vi "Offset_Gain.vi"() -> ()   [LabVIEW 2019]
uses:
  <userlib>/_TI-LA/Instr Drivers/Signal Generator/33XXX/Driver/EasyIO/Typedef/33XXX Standard Waveform Configuration.ctl
  <userlib>/_TI-LA/Instr Drivers/Signal Generator/33XXX/Driver/EasyIO/Typedef/33XXX Waveform Function.ctl
  <userlib>/_TI-LA/Instr Drivers/Signal Generator/33XXX/Driver/EasyIO/Typedef/33XXX Waveform Unit.ctl
  <userlib>/_TI-LA/Instr Drivers/Signal Generator/33XXX/Driver/EasyIO/Typedef/33XXX Output Load.ctl
  <userlib>/_TI-LA/Instr Drivers/Signal Generator/33XXX/Driver/EasyIO/Typedef/33XXX Output Load Termination.ctl
  <userlib>/_TI-LA/Instr Drivers/Signal Generator/33XXX/Driver/33XXX.lvlib
  <userlib>/_TI-LA/Instr Drivers/Signal Generator/33XXX/Modules/33XXX Modules.lvlib
  <vilib>/Analysis/NI_AALPro.lvlib
panel:
  out "intercept":dbl
  out "slope":dbl
  out "Array":dbl[](array[numeric])
  in  "lv_scomp":u16=8
  in  "lv_ref_vol":u16
  in  "lv_ref_sel":u16
  in  "Standard Waveform Configuration":T1={"Frequency (Hz)"=1000.0, "Waveform Function"=1, "DC Offset (V)"=0.0, "Unit"=0, "Amplitude (V)"=1.0, "Duty cycle (%)"=50.0} {"Duty cycle (%)" min=0.002 max=99.999 step=0.001 format="%.3p"; "Amplitude (V)" min=0.001 max=20.0 format="%#_6p"; "Unit" items=["Vpp", "Vrms", "dB"]; "DC Offset (V)" min=-10.0 max=10.0 format="%#_6p"; "Waveform Function" items=["DC", "Sine", "Square", "Triangle", "Ramp", "Pulse", "Noise", "Sinc", "Negative Ramp", "Exponential Rise", "Exponential Fall", "Cardiac"]; "Frequency (Hz)" min=1e-06 max=80000000.0 format="%#_6p"}
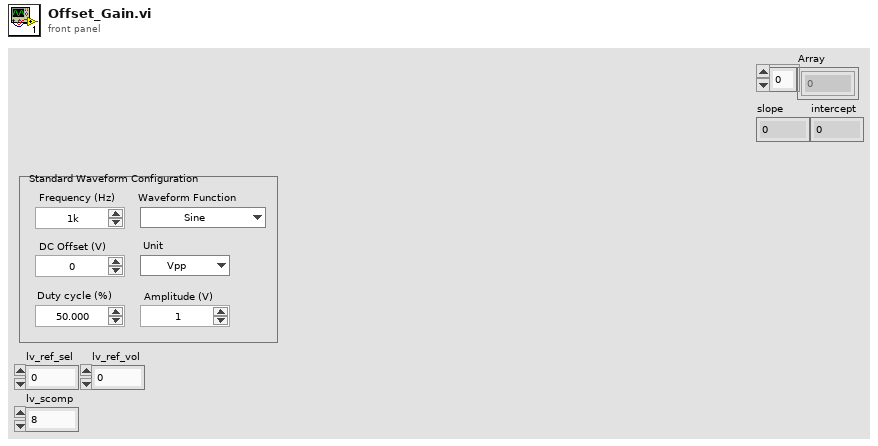
[diagram p1: front panel]
types:
  T1 = typedef "33XXX.lvlib/33XXX Standard Waveform Configuration.ctl" = cluster{"Frequency (Hz)":dbl, "Waveform Function":T2, "DC Offset (V)":dbl, "Unit":T3, "Amplitude (V)":dbl, "Duty cycle (%)":dbl}
  T2 = typedef "33XXX.lvlib/33XXX Waveform Function.ctl" = u16
  T3 = typedef "33XXX.lvlib/33XXX Waveform Unit.ctl" = u16
  T4 = typedef "33XXX.lvlib/33XXX Output Load.ctl" = cluster{"Output Load Impedence":T5, "Load value (ohms)":dbl}
  T5 = typedef "33XXX.lvlib/33XXX Output Load Termination.ctl" = enum16{"50 Ohms", "High Z", "User Defined"}
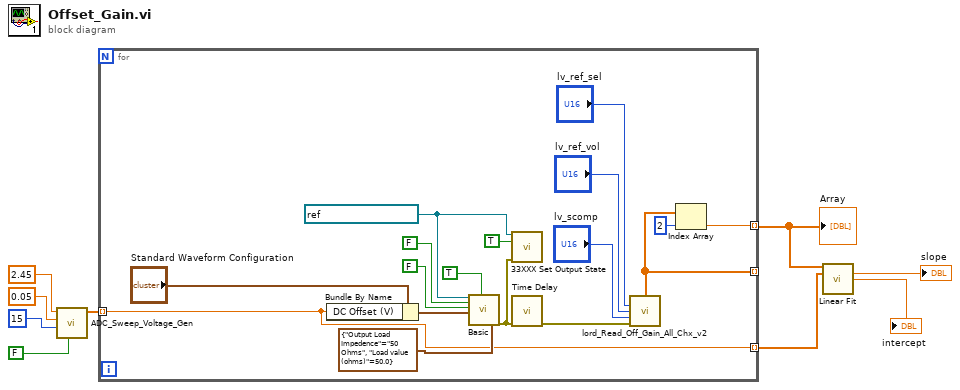
[diagram p0: block diagram]
diagram:
  n1 = call "ADC_Sweep_Voltage_Gen.vi"("Shuffle"=FALSE, "Count"=15, "Vn"=0.05, "Vp"=2.45) -> ("Vin_Array_Set"=w5:dbl[])  [unwired: 7 in]
  n2 = for {
    tunnel: w5 -> [w13] mode=indexing
    tunnel: [w13] -> w4 mode=indexing
    tunnel: [w11] -> _ mode=indexing
    tunnel: [w10] -> w3 mode=indexing
    w15 = refnum<visa-resource-name> "GPIB0::11::INSTR" ("Instrument Address")
    n3 = Bundle By Name(cluster="Standard Waveform Configuration", "DC Offset (V)"=w13) -> (w25:T1)
    n4 = call <userlib>:"Basic.vi"("Instrument Address"=w15, "Reset?"=FALSE, "ID Query?"=FALSE, "Standard Waveform Configuration"=w25, "Enable Output?"=TRUE, "Output Load Configuration"=T4 {"Output Load Impedence"=enum."50 Ohms", "Load value (ohms)"=50.0}) -> ("error out"=w16:errorcluster)  [unwired: 11 in, 2 out]
    n5 = call <userlib>:"33XXX Set Output State.vi"("VISA resource name"=w15, "Enable Output"=TRUE, "error in"=w16) -> ()  [unwired: 11 in, 2 out]
    n6 = call "Time Delay"("error in (no error)"=w16) -> ("error out"=w20:errorcluster)  [unwired: 10 in]
    n7 = call "lord_Read_Off_Gain_All_Chx_v2.vi"("lv_ref_sel"="lv_ref_sel", "lv_ref_vol"="lv_ref_vol", "lv_scomp"="lv_scomp", "error in"=w20) -> ("Mean[]"=w11:dbl[])  [unwired: 3 in, 8 out]
    n8 = Index Array(array=w11, index=2) -> (element=w10:dbl)
  }
  "Array" <- w3
  n9 = call <vilib>:"Linear Fit.vi"("Y"=w3, "X"=w4) -> ("slope"=→"slope":dbl, "intercept"=→"intercept":dbl)  [unwired: 9 in, 3 out]
